vi "Read Status Error Channel Data References.vi"(8 "error in (no error)":errorcluster, 11 "Ballard ARINC-429 Rx Execution Unit in":refnum<class "Rx Execution Unit.lvclass">) -> (0 "error out":errorcluster, 2 "status error channel data references":T2 {"specific errors"."timeout" format="%.0x"; "specific errors"."bit timing" format="%.0x"; "specific errors"."long word" format="%.0x"; "specific errors"."parity" format="%.0x"; "specific errors"."gap" format="%.0x"; "receiving" format="%.0x"}, 3 "Ballard ARINC-429 Rx Execution Unit out":refnum<class "Rx Execution Unit.lvclass">)   [LabVIEW 2020, in "AIM ARINC 429 Engine.lvlib" / "Implementation.lvlib" / "Rx Execution Unit.lvclass"]
uses:
  Rx Execution Unit.lvclass
  <vilib>/NI VeriStand/Custom Device API/Data Reference.ctl
  Rx Execution Unit.lvclass/Rx Execution Unit.ctl
  <vilib>/NI VeriStand/Custom Device API/Custom Device API.lvlib
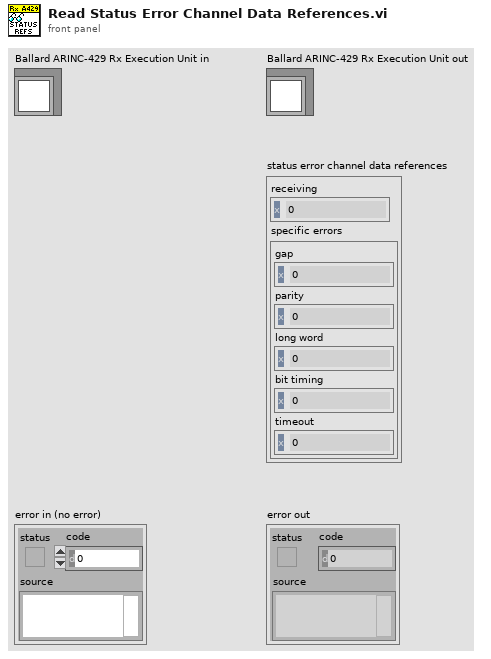
[diagram p1: front panel]
types:
  T1 = typedef "Custom Device API.lvlib/Data Reference.ctl" = i32
  T2 = cluster{"receiving":T1, "specific errors":cluster{"gap":T1, "parity":T1, "long word ":T1, "bit timing":T1, "timeout":T1}}
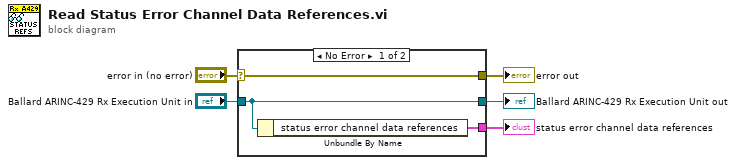
[diagram p0: block diagram]
diagram:
  n1 = case shown="No Error" "error in (no error)" {
    selector: "error in (no error)" -> [w8 w9]
    tunnel: [w8 w9] -> w4
    tunnel: [w7 w10] -> w2
    tunnel: "Ballard ARINC-429 Rx Execution Unit in" -> [w7 w10]
    tunnel: [w6 _] -> w1
    frame No Error {
      n2 = Unbundle By Name(w7) -> ("status error channel data references"=w6:T2)
    }
    frame Error {
    }
  }
  "error out" <- w4
  "Ballard ARINC-429 Rx Execution Unit out" <- w2
  "status error channel data references" <- w1
